vi "traj_coe_write_CPT_final_twomotor.vi"() -> ()   [LabVIEW 2014]
uses:
  <vilib>/Utility/file.llb/Read From Spreadsheet File (DBL).vi
  <vilib>/FPGAPlugInAG/cRIO-9066/niLvFpga_Open_cRIO-9066.vi
  <vilib>/Utility/error.llb/Error Cluster From Error Code.vi
  <vilib>/rvi/errors/niLvFpgaAdjustHostInterfaceError.vi
  <vilib>/rvi/interface/nirviOpenFPGA/nirviOpenFPGA.xnode
  FPGA Bitfiles/forcecontroledu_FPGATarget_impedufinaltwomo_3w-fwrV9O4Q.lvbitx
  FPGA VIs/imp_edu_final_twomotor_pid.vi
  <vilib>/rvi/interface/nirviMethod/nirviMethod.xnode
  <vilib>/FPGAPlugInAG/cRIO-9066/niLvFpga_WriteFifo_cRIO-9066.vi
  <vilib>/rvi/errors/niLvFpgaMergeErrorWithErrorCode.vi
panel:
  out "A3_y":dbl[](array[numeric]) format="%.2f"
  out "A1_y":dbl[](array[numeric]) format="%.2f"
  out "A2_y":dbl[](array[numeric]) format="%.2f"
  out "A0_y":dbl[](array[numeric]) format="%.2f"
  out "A3_p":dbl[](array[numeric]) format="%.2f"
  out "writing_done":bool
  in  "stop":bool
  out "A1_p":dbl[](array[numeric]) format="%.2f"
  out "A2_p":dbl[](array[numeric]) format="%.2f"
  out "A0_p":dbl[](array[numeric]) format="%.2f"
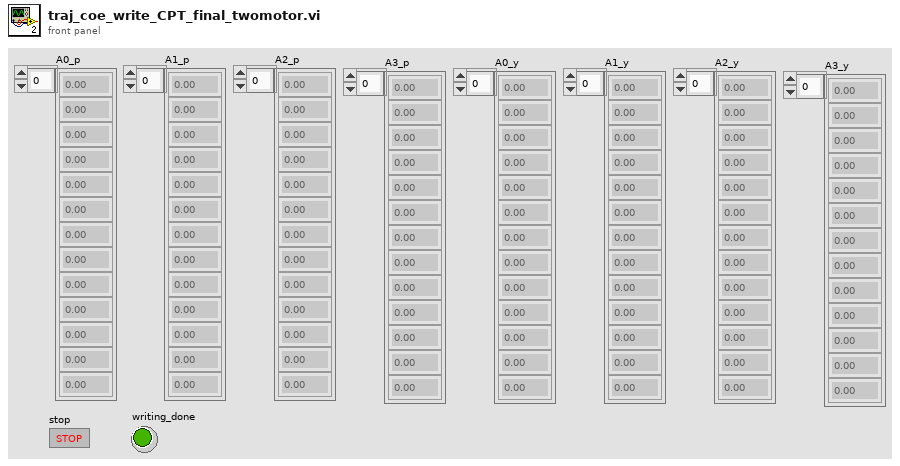
[diagram p1: front panel]
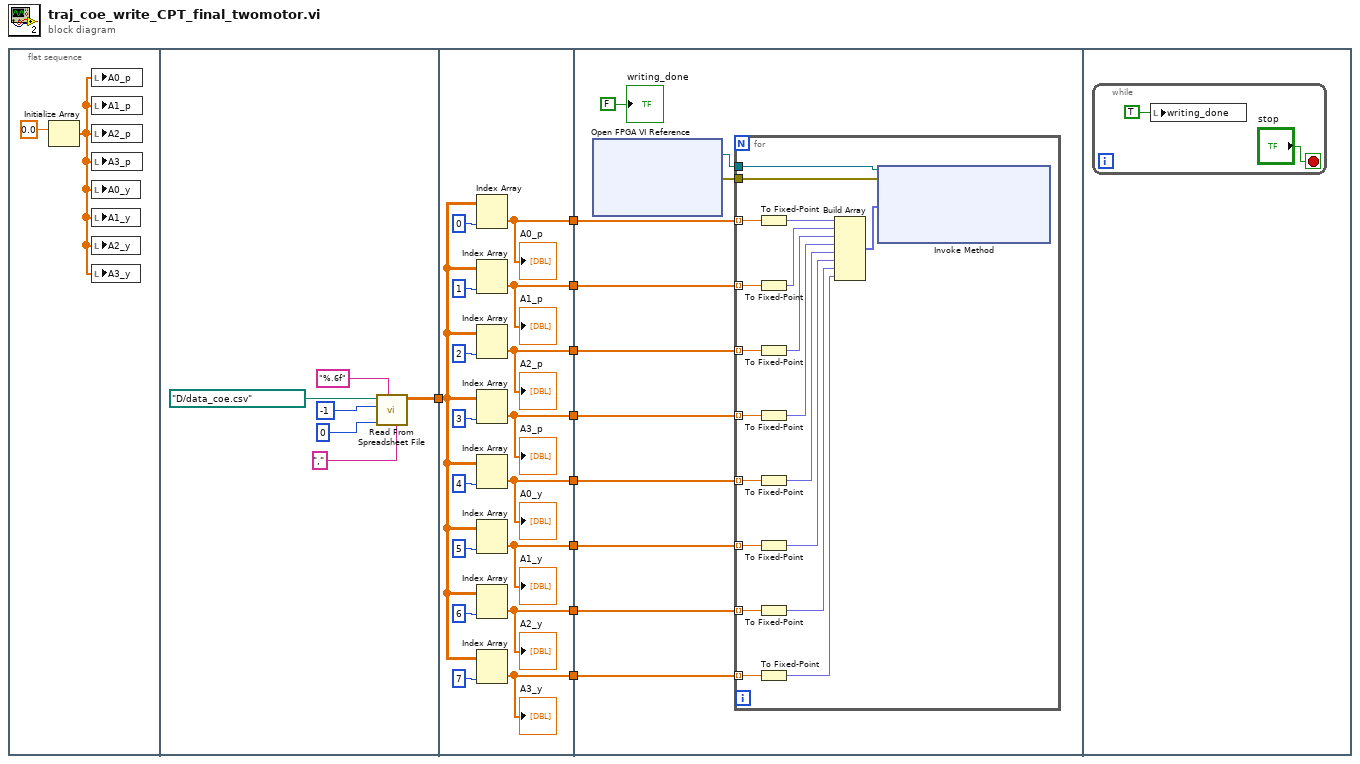
[diagram p0: block diagram]
diagram:
  n1 = flat-sequence {
    tunnel: [w12] -> w9
    tunnel: w9 -> [w22]
    tunnel: [w31] -> w8
    tunnel: [w30] -> w7
    tunnel: [w29] -> w6
    tunnel: [w27] -> w5
    tunnel: [w21] -> w4
    tunnel: [w20] -> w3
    tunnel: [w19] -> w2
    tunnel: [w18] -> w1
    tunnel: w8 -> [w45]
    tunnel: w7 -> [w44]
    tunnel: w6 -> [w43]
    tunnel: w5 -> [w41]
    tunnel: w4 -> [w38]
    tunnel: w3 -> [w37]
    tunnel: w2 -> [w36]
    tunnel: w1 -> [w35]
    frame #0 {
      n2 = Initialize Array(0.0 ("element")) -> (w10:dbl[])  [unwired: 1 in]
      n3 = local write "A0_p"(w10) -> ()
      n4 = local write "A1_p"(w10) -> ()
      n5 = local write "A2_p"(w10) -> ()
      n6 = local write "A3_p"(w10) -> ()
      n7 = local write "A0_y"(w10) -> ()
      n8 = local write "A1_y"(w10) -> ()
      n9 = local write "A2_y"(w10) -> ()
      n10 = local write "A3_y"(w10) -> ()
    }
    frame #1 {
      n11 = call-poly <vilib>:"Read From Spreadsheet File.vi"("delimiter (\\t)"="," ("delimiter (\\t)"), "format (%.3f)"="%.6f" ("format (%d)"), "max characters/row  (no limit:0)"=0, "number of rows (all:-1)"=-1, "file path (dialog if empty)"=path "D:/data_coe.csv") -> ("all rows"=w12:dbl[][])  [unwired: 2 in, 4 out]
    }
    frame #2 {
      n12 = Index Array(array=w22, index (col)=0 ("disabled index (col)")) -> (element=w31:dbl[])  [unwired: 1 in]
      "A0_p" <- w31
      n13 = Index Array(array=w22, index (col)=1 ("disabled index (col)")) -> (element=w30:dbl[])  [unwired: 1 in]
      "A1_p" <- w30
      n14 = Index Array(array=w22, index (col)=2 ("disabled index (col)")) -> (element=w29:dbl[])  [unwired: 1 in]
      "A2_p" <- w29
      n15 = Index Array(array=w22, index (col)=3 ("disabled index (col)")) -> (element=w27:dbl[])  [unwired: 1 in]
      "A3_p" <- w27
      n16 = Index Array(array=w22, index (col)=4) -> (element=w21:dbl[])  [unwired: 1 in]
      "A0_y" <- w21
      n17 = Index Array(array=w22, index (col)=5) -> (element=w20:dbl[])  [unwired: 1 in]
      "A1_y" <- w20
      n18 = Index Array(array=w22, index (col)=6) -> (element=w19:dbl[])  [unwired: 1 in]
      "A2_y" <- w19
      n19 = Index Array(array=w22, index (col)=7) -> (element=w18:dbl[])  [unwired: 1 in]
      "A3_y" <- w18
    }
    frame #3 {
      n20 = xnode "Open FPGA VI Reference"() -> ("FPGA VI Reference Out"=w40:refnum<k20>, "error out"=w39:errorcluster)  [unwired: 2 in]
      n21 = for {
        tunnel: w40 -> [w56]
        tunnel: w39 -> [w55]
        tunnel: w45 -> [w64] mode=indexing
        tunnel: w44 -> [w63] mode=indexing
        tunnel: w43 -> [w62] mode=indexing
        tunnel: w41 -> [w58] mode=indexing
        tunnel: w38 -> [w49] mode=indexing
        tunnel: w37 -> [w48] mode=indexing
        tunnel: w36 -> [w47] mode=indexing
        tunnel: w35 -> [w46] mode=indexing
        n22 = To Fixed-Point(number=w64) -> (fixed-point=w61:fxp<+/-,30,15>)  [unwired: 1 in]
        n23 = To Fixed-Point(number=w63) -> (fixed-point=w60:fxp<+/-,30,15>)  [unwired: 1 in]
        n24 = To Fixed-Point(number=w62) -> (fixed-point=w59:fxp<+/-,30,15>)  [unwired: 1 in]
        n25 = To Fixed-Point(number=w58) -> (fixed-point=w57:fxp<+/-,30,15>)  [unwired: 1 in]
        n26 = To Fixed-Point(number=w49) -> (fixed-point=w53:fxp<+/-,30,15>)  [unwired: 1 in]
        n27 = To Fixed-Point(number=w48) -> (fixed-point=w52:fxp<+/-,30,15>)  [unwired: 1 in]
        n28 = To Fixed-Point(number=w47) -> (fixed-point=w51:fxp<+/-,30,15>)  [unwired: 1 in]
        n29 = To Fixed-Point(number=w46) -> (fixed-point=w50:fxp<+/-,30,15>)  [unwired: 1 in]
        n30 = Build Array(w61, w60, w59, w57, w53, w52, w51, w50) -> (w54:fxp<+/-,30,15>[])
        n31 = xnode "Invoke Method"("FPGA VI Reference In"=w56, "error in"=w55, "Data"=w54) -> ()  [unwired: 1 in, 3 out]
      }
      "writing_done" <- FALSE ("writing_done")
    }
    frame #4 {
      n32 = while {
        stop <- "stop" stop-if-true
        n33 = local write "writing_done"(TRUE ("writing_done")) -> ()
      }
    }
  }
